vi "Acquisitions (FPGA).vi"() -> ()   [LabVIEW 2019]
uses:
  <vilib>/LabVIEW Targets/FPGA/cRIO/shared/nicrio_ModuleControls/nicrio_cRIO-9775_ContinuousDataRates4ChansRing.ctl
  <vilib>/LabVIEW Targets/FPGA/cRIO/shared/nicrio_ModuleControls/nicrio_BasicConversionTime.ctl
  <vilib>/rvi/Emulation/niFpgaGetClockAttributes.vi
  <vilib>/rvi/Emulation/niFpgaSctlEmulationGetInTimedLoop.vi
  <vilib>/rvi/Emulation/niFpgaEmulationReportErrorSimple.vi
  <vilib>/rvi/eio/common/nirviEmuTemplatePropertySet_errors.vi
  <vilib>/rvi/eio/common/nirviEmuTemplateMethod_errors.vi
  <vilib>/rvi/interface/RandomDataEmulation/niFpgaRandomDataHandleErrors.vi
  <vilib>/rvi/Emulation/niFpgaCriticalErrorInLSC.vi
  <vilib>/rvi/Emulation/niFpgaProcessEmulError.vi
  <vilib>/eio/EIOPropertyNode/EIOPropertyNode.xnode
  <vilib>/eio/EIONode/EIONode.xnode
  <vilib>/rvi/DataTransferAndStorage/Container/XNode/niFpgaContainer.xnode
  <vilib>/rvi/interface/RandomDataEmulation/nirviRandomDataFpgaReadWriteTemplate.vi
  <vilib>/rvi/eio/common/nirviEmuTemplatePropertyGet_errors.vi
  <vilib>/rvi/eio/common/nirviEmuTemplatePropertyGet_noerrors.vi
  <vilib>/rvi/eio/common/nirviEmuTemplatePropertySet_noerrors.vi
panel:
  out "appended array 2":fxp<+/-,17,5>[](array[numeric])
  out "appended array":fxp<+/-,20,5>[](array[numeric])
  in  "Timing Mode":T1
  in  "Continuous Data Rate":T2=20 items=["1.000 MS/s (NI 9775)"=20, "833.333 KS/s (NI 9775)"=24, "714.286 KS/s (NI 9775)"=28, "625.000 KS/s (NI 9775)"=32, "555.556 KS/s (NI 9775)"=36, "500.000 KS/s (NI 9775)"=40, "454.545 KS/s (NI 9775)"=44, "416.667 KS/s (NI 9775)"=48, "384.615 KS/s (NI 9775)"=52, "357.143 KS/s (NI 9775)"=56, "333.333 KS/s (NI 9775)"=60, "312.500 KS/s (NI 9775)"=64, "294.118 KS/s (NI 9775)"=68, "277.778 KS/s (NI 9775)"=72, "263.158 KS/s (NI 9775)"=76, "250.000 KS/s (NI 9775)"=80, "238.095 KS/s (NI 9775)"=84, "227.273 KS/s (NI 9775)"=88, "217.391 KS/s (NI 9775)"=92, "208.333 KS/s (NI 9775)"=96, "200.000 KS/s (NI 9775)"=100, "192.308 KS/s (NI 9775)"=104, "185.185 KS/s (NI 9775)"=108, "178.571 KS/s (NI 9775)"=112, "172.414 KS/s (NI 9775)"=116, "166.667 KS/s (NI 9775)"=120, "161.290 KS/s (NI 9775)"=124, "156.250 KS/s (NI 9775)"=128, "151.515 KS/s (NI 9775)"=132, "147.059 KS/s (NI 9775)"=136, "142.857 KS/s (NI 9775)"=140, "138.889 KS/s (NI 9775)"=144, "135.135 KS/s (NI 9775)"=148, "131.579 KS/s (NI 9775)"=152, "128.205 KS/s (NI 9775)"=156, "125.000 KS/s (NI 9775)"=160, "121.951 KS/s (NI 9775)"=164, "119.048 KS/s (NI 9775)"=168, "116.279 KS/s (NI 9775)"=172, "113.636 KS/s (NI 9775)"=176, "111.111 KS/s (NI 9775)"=180, "108.696 KS/s (NI 9775)"=184, "106.383 KS/s (NI 9775)"=188, "104.167 KS/s (NI 9775)"=192, "102.041 KS/s (NI 9775)"=196, "100.000 KS/s (NI 9775)"=200, "50.000 KS/s (NI 9775)"=400, "33.333 KS/s (NI 9775)"=600, "25.000 KS/s (NI 9775)"=800, "20.000 KS/s (NI 9775)"=1000, "16.667 KS/s (NI 9775)"=1200, "14.286 KS/s (NI 9775)"=1400, "12.500 KS/s (NI 9775)"=1600, "11.111 KS/s (NI 9775)"=1800, "10.000 KS/s (NI 9775)"=2000, "9.091 KS/s (NI 9775)"=2200, "8.333 KS/s (NI 9775)"=2400, "7.692 KS/s (NI 9775)"=2600, "7.143 KS/s (NI 9775)"=2800, "6.667 KS/s (NI 9775)"=3000, "6.250 KS/s (NI 9775)"=3200, "5.882 KS/s (NI 9775)"=3400, "5.556 KS/s (NI 9775)"=3600, "5.000 KS/s (NI 9775)"=4000, "4.762 KS/s (NI 9775)"=4200, "4.545 KS/s (NI 9775)"=4400, "4.348 KS/s (NI 9775)"=4600, "4.167 KS/s (NI 9775)"=4800, "4.000 KS/s (NI 9775)"=5000, "3.846 KS/s (NI 9775)"=5200, "3.571 KS/s (NI 9775)"=5600, "3.333 KS/s (NI 9775)"=6000, "3.125 KS/s (NI 9775)"=6400, "2.941 KS/s (NI 9775)"=6800, "2.778 KS/s (NI 9775)"=7200, "2.632 KS/s (NI 9775)"=7600, "2.500 KS/s (NI 9775)"=8000, "2.381 KS/s (NI 9775)"=8400, "2.273 KS/s (NI 9775)"=8800, "2.174 KS/s (NI 9775)"=9200, "2.083 KS/s (NI 9775)"=9600, "2.000 KS/s (NI 9775)"=10000, "1.923 KS/s (NI 9775)"=10400, "1.852 KS/s (NI 9775)"=10800, "1.786 KS/s (NI 9775)"=11200, "1.724 KS/s (NI 9775)"=11600, "1.667 KS/s (NI 9775)"=12000, "1.613 KS/s (NI 9775)"=12400, "1.563 KS/s (NI 9775)"=12800, "1.515 KS/s (NI 9775)"=13200, "1.471 KS/s (NI 9775)"=13600, "1.429 KS/s (NI 9775)"=14000, "1.389 KS/s (NI 9775)"=14400, "1.351 KS/s (NI 9775)"=14800, "1.316 KS/s (NI 9775)"=15200, "1.282 KS/s (NI 9775)"=15600, "1.250 KS/s (NI 9775)"=16000, "1.220 KS/s (NI 9775)"=16400, "1.190 KS/s (NI 9775)"=16800, "1.163 KS/s (NI 9775)"=17200, "1.136 KS/s (NI 9775)"=17600, "1.111 KS/s (NI 9775)"=18000, "1.087 KS/s (NI 9775)"=18400, "1.064 KS/s (NI 9775)"=18800, "1.042 KS/s (NI 9775)"=19200, "1.020 KS/s (NI 9775)"=19600, "1.000 KS/s (NI 9775)"=20000, "0.980 KS/s (NI 9775)"=20400, "0.962 KS/s (NI 9775)"=20800, "0.943 KS/s (NI 9775)"=21200, "0.926 KS/s (NI 9775)"=21600, "0.909 KS/s (NI 9775)"=22000, "0.893 KS/s (NI 9775)"=22400, "0.877 KS/s (NI 9775)"=22800, "0.862 KS/s (NI 9775)"=23200, "0.847 KS/s (NI 9775)"=23600, "0.833 KS/s (NI 9775)"=24000, "0.820 KS/s (NI 9775)"=24400, "0.806 KS/s (NI 9775)"=24800, "0.794 KS/s (NI 9775)"=25200, "0.781 KS/s (NI 9775)"=25600, "0.694 KS/s (NI 9775)"=28800, "0.625 KS/s (NI 9775)"=32000, "0.568 KS/s (NI 9775)"=35200, "0.521 KS/s (NI 9775)"=38400, "0.446 KS/s (NI 9775)"=44800, "0.391 KS/s (NI 9775)"=51200, "0.347 KS/s (NI 9775)"=57600, "0.313 KS/s (NI 9775)"=64000]
  out "Data FIFO Full":bool
  in  "Stop":bool
  in  "Loop Rate 9215 (uS)":u32
  out "Data2 FIFO Full":bool
  out "FPGA Error Out":errorcluster
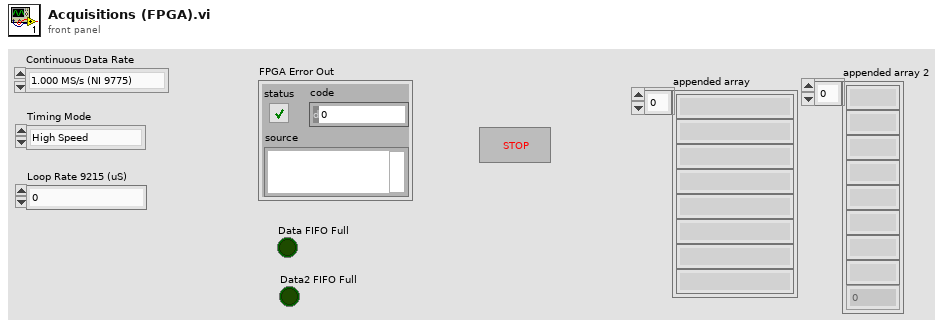
[diagram p1: front panel]
types:
  T1 = typedef "nicrio_BasicConversionTime.ctl" = enum8{"High Speed", "High Resolution"}
  T2 = typedef "nicrio_cRIO-9775_ContinuousDataRates4ChansRing.ctl" = u16
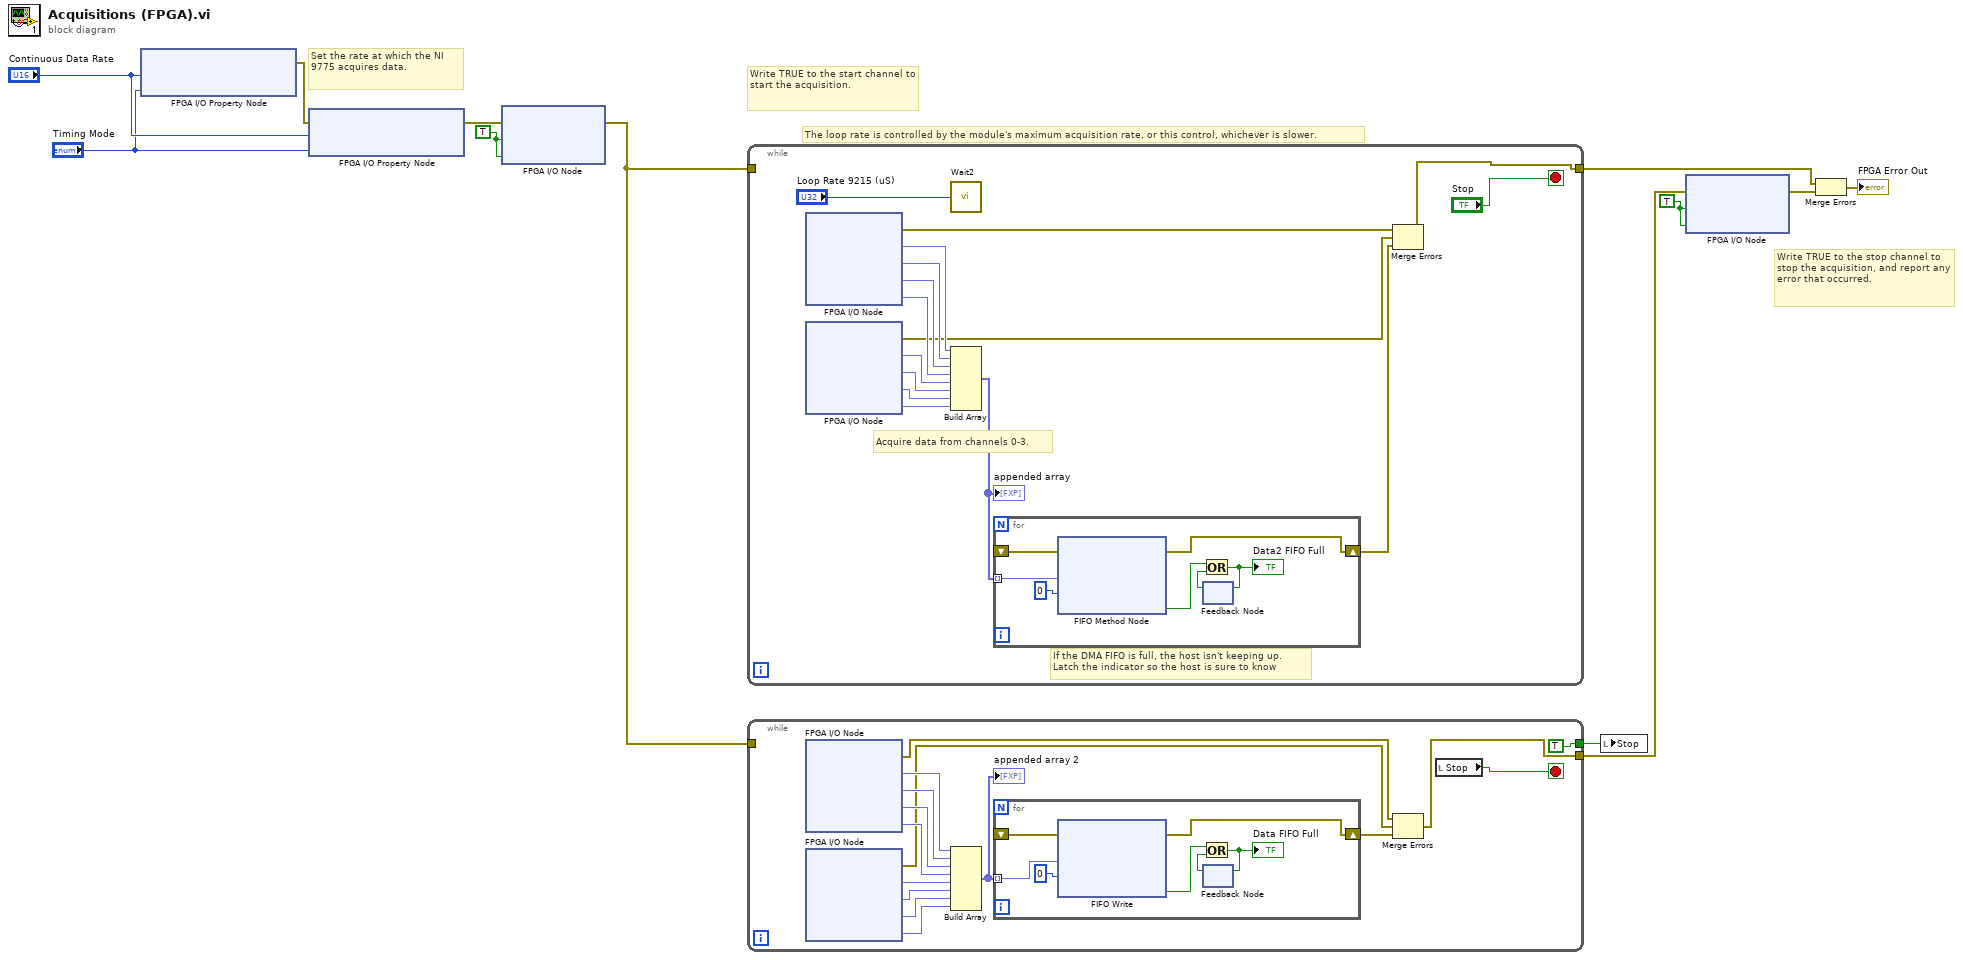
[diagram p0: block diagram]
diagram:
  w9 = TRUE
  w4 = TRUE
  # "Write TRUE to the stop channel to stop the acquisition, and report any error that occurred."
  # "Write TRUE to the start channel to start the acquisition."
  # "Set the rate at which the NI 9775 acquires data."
  # "The loop rate is controlled by the module's maximum acquisition rate, or this control, whichever is slower."
  n1 = xnode "FPGA I/O Property Node"("Continuous Data Rate"="Continuous Data Rate", "Timing Mode"="Timing Mode") -> ("error out"=w8:errorcluster)  [unwired: 2 in, 1 out]
  n2 = xnode "FPGA I/O Property Node"("error in"=w8, "Continuous Data Rate"="Continuous Data Rate", "Timing Mode"="Timing Mode") -> ("error out"=w7:errorcluster)  [unwired: 1 in, 1 out]
  n3 = xnode "FPGA I/O Node"("error in"=w7, "Mod1/Start"=w9, "Mod2/Start"=w9) -> ("error out"=w1:errorcluster)  [unwired: 2 in, 2 out]
  n4 = while {
    tunnel: [w13] -> w12
    tunnel: w1 -> [_]
    stop <- "Stop" stop-if-true
    # "Acquire data from channels 0-3."
    # "If the DMA FIFO is full, the host isn't keeping up. \nLatch the indicator so the host is sure to know"
    n5 = xnode "FPGA I/O Node"() -> ("error out"=w20:errorcluster, "Mod3/AI0"=w25:fxp<+/-,20,5>, "Mod3/AI1"=w24:fxp<+/-,20,5>, "Mod3/AI2"=w23:fxp<+/-,20,5>, "Mod3/AI3"=w22:fxp<+/-,20,5>)  [unwired: 5 in, 4 out]
    n6 = xnode "FPGA I/O Node"() -> ("error out"=w15:errorcluster, "Mod4/AI0"=w19:fxp<+/-,20,5>, "Mod4/AI1"=w18:fxp<+/-,20,5>, "Mod4/AI2"=w17:fxp<+/-,20,5>, "Mod4/AI3"=w16:fxp<+/-,20,5>)  [unwired: 5 in, 4 out]
    n7 = call "Wait2"("Count(uSec)"="Loop Rate 9215 (uS)") -> ()  [unwired: 1 out]
    n8 = Build Array(w25, w24, w23, w22, w19, w18, w17, w16) -> (w26:fxp<+/-,20,5>[])
    "appended array" <- w26
    n9 = for {
      tunnel: w26 -> [w34] mode=indexing
      shift-right: [w29] -> w14
      shift-left: _ -> [w28]
      n10 = xnode ("FIFO Method Node")("Element"=w34, "Timeout"=0, "error in (no error)"=w28) -> ("Timed Out?"=w30:bool, "error out"=w29:errorcluster)  [unwired: 1 in, 1 out]
      n11 = feedback #1() -> (w32:bool)  [unwired: 1 out]
      n12 = Or(x=w30, y=w32) -> (x .or. y?=w31:bool)
      "Data2 FIFO Full" <- w31
      n13 = feedback-in #1(w31) -> ()
    }
    n14 = Merge Errors(w20, w15, w14) -> (w13:errorcluster)
  }
  n15 = while {
    tunnel: w1 -> [_]
    tunnel: [w38] -> w10
    tunnel: [TRUE ("Stop")] -> w2
    stop <- w43 stop-if-true
    n16 = xnode "FPGA I/O Node"() -> ("error out"=w45:errorcluster, "Mod1/AI0"=w49:fxp<+/-,17,5>, "Mod1/AI1"=w48:fxp<+/-,17,5>, "Mod1/AI2"=w47:fxp<+/-,17,5>, "Mod1/AI3"=w46:fxp<+/-,17,5>)  [unwired: 5 in, 4 out]
    n17 = xnode "FPGA I/O Node"() -> ("error out"=w37:errorcluster, "Mod2/AI0"=w42:fxp<+/-,17,5>, "Mod2/AI1"=w41:fxp<+/-,17,5>, "Mod2/AI2"=w40:fxp<+/-,17,5>, "Mod2/AI3"=w39:fxp<+/-,17,5>)  [unwired: 5 in, 4 out]
    n18 = Build Array(w49, w48, w47, w46, w42, w41, w40, w39) -> (w35:fxp<+/-,17,5>[])
    "appended array 2" <- w35
    n19 = for {
      tunnel: w35 -> [w53] mode=indexing
      shift-right: [w50] -> w36
      shift-left: _ -> [w51]
      n20 = xnode ("FIFO Write")("Element"=w53, "Timeout"=0 ("Timeout (-1 for no timeout)"), "error in (no error)"=w51) -> ("Timed Out?"=w54:bool, "error out"=w50:errorcluster)  [unwired: 1 in, 1 out]
      n21 = feedback #2() -> (w55:bool)  [unwired: 1 out]
      n22 = Or(x=w54, y=w55) -> (x .or. y?=w56:bool)
      "Data FIFO Full" <- w56
      n23 = feedback-in #2(w56) -> ()
    }
    n24 = Merge Errors(w45, w37, w36) -> (w38:errorcluster)
    n25 = local read "Stop"() -> (w43:bool)
  }
  n26 = local write "Stop"(w2) -> ()
  n27 = xnode "FPGA I/O Node"("error in"=w10, "Mod1/Stop"=w4, "Mod2/Stop"=w4) -> ("error out"=w3:errorcluster)  [unwired: 2 in, 2 out]
  n28 = Merge Errors(w12, w3) -> (→"FPGA Error Out":errorcluster)
